vi "SerializeMetadataToJson.vi"(8 "error in (no error)":errorcluster, 11 "head in":refnum<data-value>) -> (0 "error out":errorcluster, 2 "Serialized String":string, 3 "head out":refnum<data-value>)   [LabVIEW 2017, in "DirectoryMetadata.lvclass"]
uses:
  DirectoryMetadata.lvclass
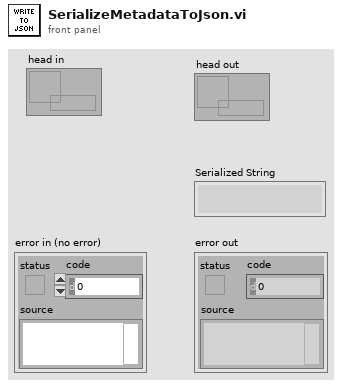
[diagram p1: front panel]
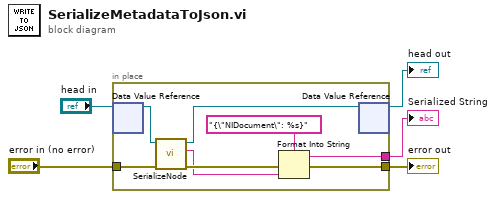
[diagram p0: block diagram]
diagram:
  n1 = in-place {
    in-place-border: "error in (no error)" -> [w13]
    in-place-border: [w8] -> w4
    in-place-border: [w9] -> w3
    n2 = in-place-dvr #1("head in") -> (w11:refnum<class "DirectoryMetadata.lvclass">)  [unwired: 1 out]
    n3 = call "SerializeNode.vi"("error in (no error)"=w13, "Node in"=w11) -> ("error out"=w12:errorcluster, "Serialized String"=w6:string, "Node out"=w10:refnum<class "DirectoryMetadata.lvclass">)  [unwired: 7 in]
    n4 = Format Into String(format string="{\"NIDocument\": %s}", error in=w12, w6) -> (resulting string=w8:string, error out=w9:errorcluster)  [unwired: 1 in]
    n5 = in-place-dvr #1(w10) -> (→"head out":refnum<data-value>)  [unwired: 1 out]
  }
  "Serialized String" <- w4
  "error out" <- w3
